vi "Facade.vi"(0 "Data In":T8={"Name"="", "Criteria"=[{"DigInput"=0, "State"=enum."Low", "Time (ms)"=0, "Name"=""}, {"DigInput"=0, "State"=enum."Low", "Time (ms)"=0, "Name"=""}], "Operators"=[], "Accumulator"={"active"=FALSE, "N"=0, "T"=0.0, "Imax"=0.0, "latency"=0.0}}, 2 "Display State In":T6, 3 "Container State":T7) -> (6 "Data Out":T8={"Name"="", "Criteria"=[{"DigInput"=0, "State"=enum."Low", "Time (ms)"=0, "Name"=""}, {"DigInput"=0, "State"=enum."Low", "Time (ms)"=0, "Name"=""}], "Operators"=[], "Accumulator"={"active"=FALSE, "N"=0, "T"=0.0, "Imax"=0.0, "latency"=0.0}}, 7 "Display State Out":T6, 8 "Action":T5)   [LabVIEW 2020, in "Input Event XCtrl.xctl"]
uses:
  Input Event XCtrl.xctl
  <vilib>/_xctls/Action.ctl
  <vilib>/_xctls/XControlSupport.lvlib
  Input Criteria Table/Input Criteria Table.xctl
  <vilib>/_xctls/Container State.ctl
  Data.vi
  State.vi
  epl-vi-lib/Utility VIs/Type Defs/Logic State.ctl
  Digital Input VIs/Tosca-Input Criterion.ctl
  Typedefs/Tosca-Accumulator.ctl
  epl-vi-lib/Utility VIs/Buttons/KCheckmarkBoolean 2.ctl
panel:
  in  "label1":string="...beginning"
  in  "label2":string="...no interval longer than"
  in  "latency":dbl caption="ms after state change..."
  in  "ms":dbl
  in  "T":dbl caption="ms..."
  in  "N":i32=2 caption="in" min=2
  in  "Accumulate":T1
  in  "Input Criteria":T4(xcontrol) caption="...is TRUE when..."
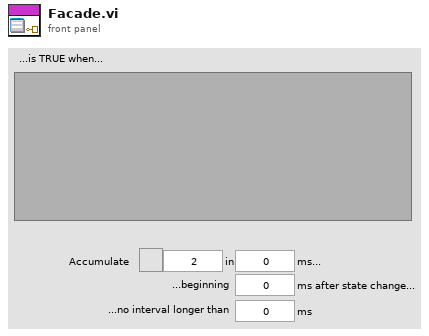
[diagram p1: front panel]
types:
  T1 = typedef "KCheckmarkBoolean 2.ctl" = bool
  T2 = typedef "Tosca-Input Criterion.ctl" = cluster{"DigInput":i32, "State":T3, "Time (ms)":i32, "Name":string}
  T3 = typedef "Logic State.ctl" = enum16{"Low", "High", "Rising", "Falling"}
  T4 = cluster{"Name":string, "Criteria":T2[], "Operators":enum16{"AND", "OR"}[]}
  T5 = typedef "XControlSupport.lvlib/Action.ctl" = cluster{"Data Changed?":bool, "State Changed?":bool, "Action Name":string}
  T6 = typedef "Input Event XCtrl.xctl/State.vi" = cluster{"Digital Inputs":string[], "Flags":string[], "action":string}
  T7 = typedef "XControlSupport.lvlib/Container State.ctl" = cluster{"Indicator?":bool, "Run Mode?":bool, " Refnum":refnum<vi>}
  T8 = typedef "Input Event XCtrl.xctl/Data.vi" = cluster{"Name":string, "Criteria":T2[], "Operators":enum16{"AND", "OR"}[], "Accumulator":T9}
  T9 = typedef "Tosca-Accumulator.ctl" = cluster{"active":bool, "N":i32, "T":dbl, "Imax":dbl, "latency":dbl}
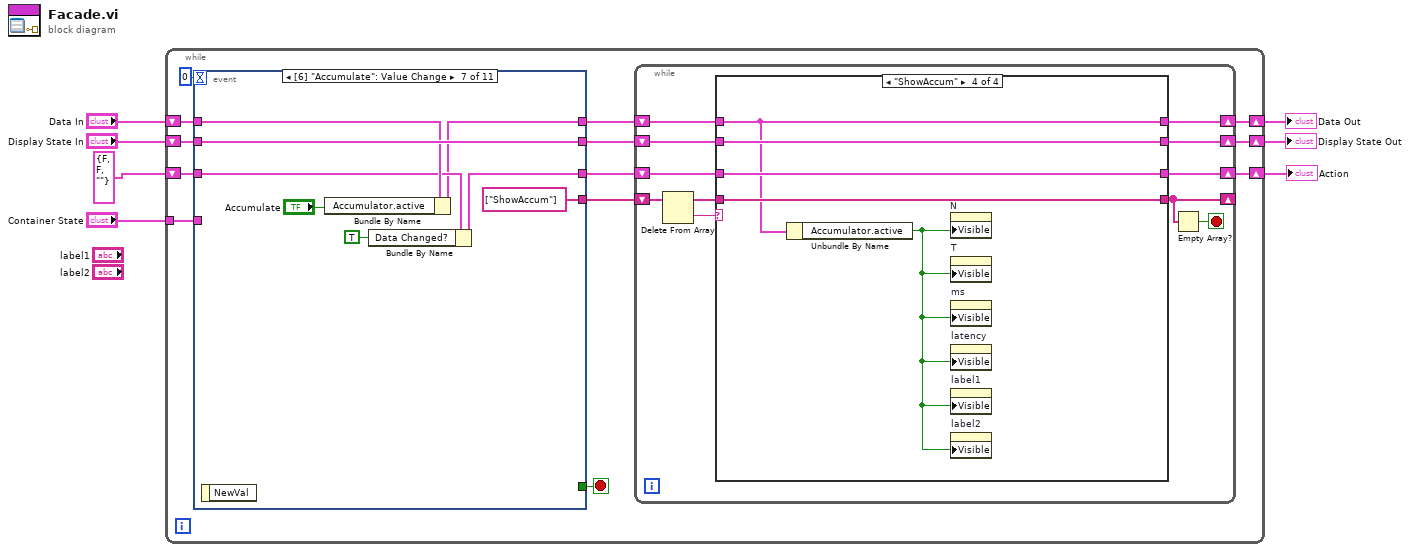
[diagram p0: block diagram]
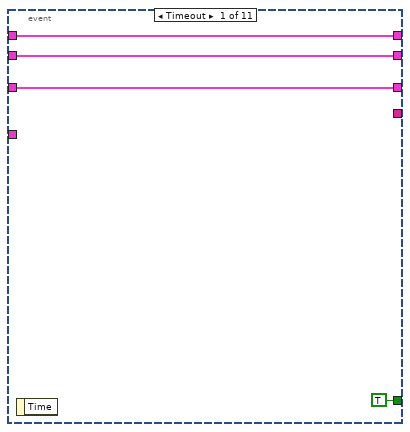
[diagram p2: hidden frame]
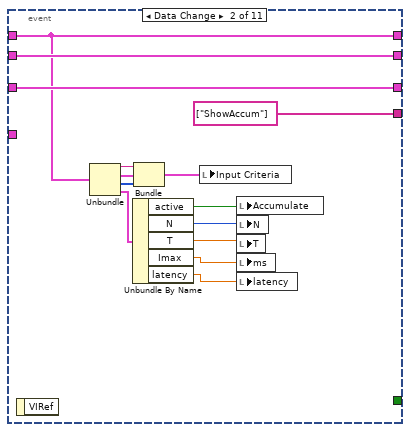
[diagram p3: hidden frame]
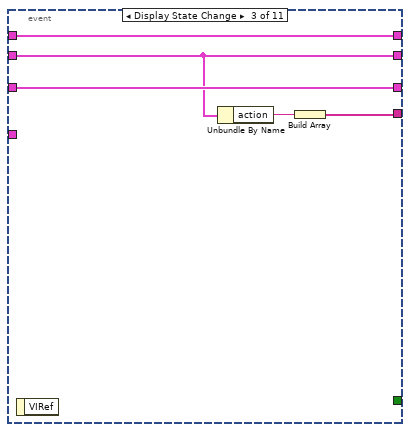
[diagram p4: hidden frame]
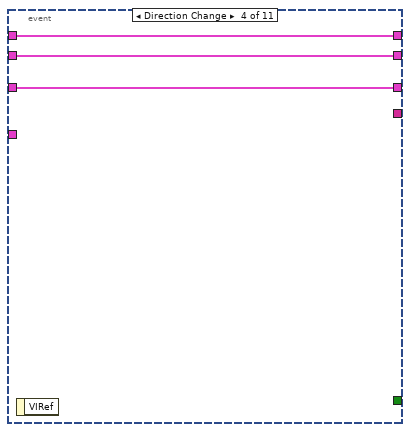
[diagram p5: hidden frame]
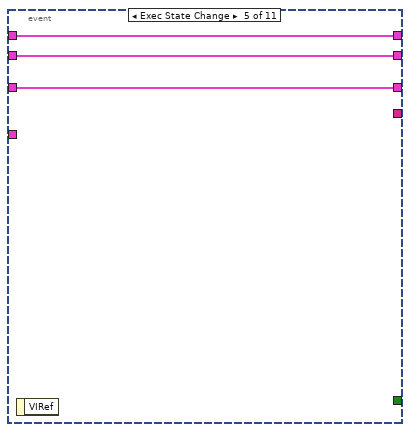
[diagram p6: hidden frame]
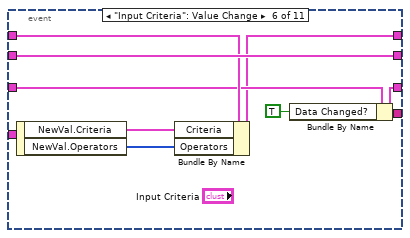
[diagram p7: hidden frame]
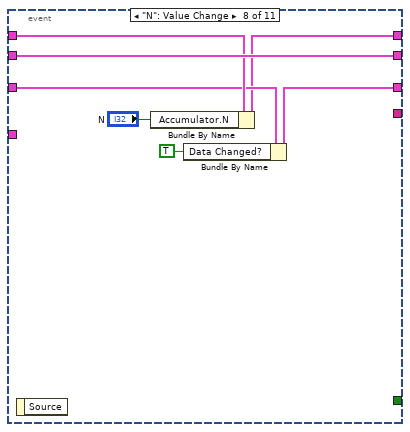
[diagram p8: hidden frame]
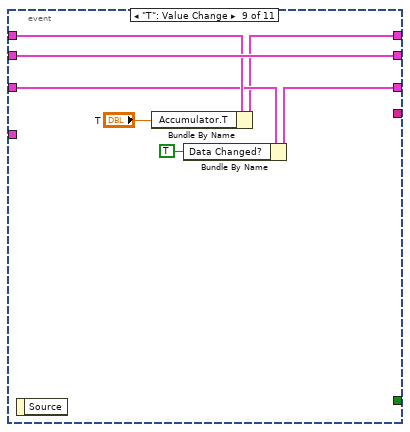
[diagram p9: hidden frame]
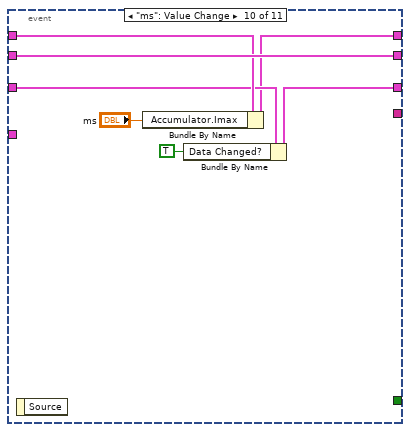
[diagram p10: hidden frame]
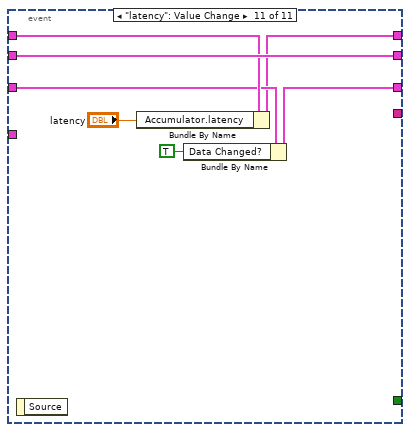
[diagram p11: hidden frame]
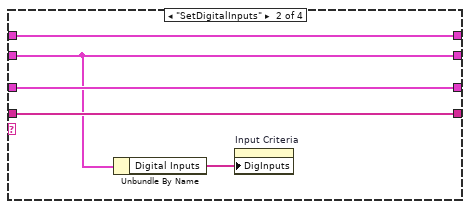
[diagram p13: hidden frame]
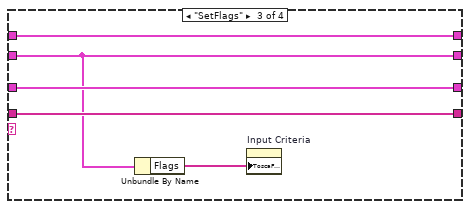
[diagram p14: hidden frame]
diagram:
  n1 = while {
    shift-right: [w8] -> w4
    shift-left: "Display State In" -> [w20]
    tunnel: "Container State" -> [w17]
    shift-right: [w10] -> w7
    shift-left: "Data In" -> [w16]
    shift-right: [w9] -> w2
    shift-left: T5 {"Data Changed?"=FALSE, "State Changed?"=FALSE, "Action Name"=""} ("Action") -> [w15]
    stop <- w19 stop-if-true
    n2 = event shown="[6] \"Accumulate\": Value Change" {
      selector: _ -> [_ _ _ _ _ _ _ _ _ _ _]
      dyn-events: _ -> [_ _ _ _ _ _ _ _ _ _ _]
      timeout: 0 -> [_ _ _ _ _ _ _ _ _ _ _]
      tunnel: w20 -> [w22 w38 w41 w46 w49 w57 w65 w72 w79 w86 w93]
      tunnel: [w22 w38 w41 w46 w49 w57 w65 w72 w79 w86 w93] -> w12
      tunnel: [TRUE _ _ _ _ _ _ _ _ _ _] -> w19
      tunnel: w17 -> [_ _ _ _ _ _ _ _ _ _ _]
      tunnel: w16 -> [w21 w31 w43 w45 w48 w56 w64 w71 w78 w85 w92]
      tunnel: [w21 w31 w43 w45 w48 w54 w61 w69 w76 w83 w90] -> w13
      tunnel: [w23 w37 w42 w44 w47 w53 w60 w68 w75 w82 w89] -> w11
      tunnel: w15 -> [w23 w37 w42 w44 w47 w55 w63 w70 w77 w84 w91]
      tunnel: [_ string[] ["ShowAccum"] w39 _ _ _ string[] ["ShowAccum"] _ _ _ _] -> w14
      event Timeout {
        n3 = event-data() -> ()  [unwired: 1 in, 1 out]
      }
      event Data Change {
        n4 = event-data() -> ()  [unwired: 1 in, 1 out]
        n5 = Unbundle(w31) -> ("Name"=w35:string, "Criteria"=w34:T2[], "Operators"=w33:enum16{"AND", "OR"}[], "Accumulator"=w32:T9)
        n6 = Unbundle By Name(w32) -> ("active"=w29:bool, "N"=w28:i32, "T"=w27:dbl, "Imax"=w26:dbl, "latency"=w25:dbl)
        n7 = Bundle("Name"=w35, "Criteria"=w34, "Operators"=w33) -> (w30:T4)  [unwired: 1 in]
        n8 = local write "Input Criteria"(w30) -> ()
        n9 = local write "Accumulate"(w29) -> ()
        n10 = local write "N"(w28) -> ()
        n11 = local write "T"(w27) -> ()
        n12 = local write "ms"(w26) -> ()
        n13 = local write "latency"(w25) -> ()
      }
      event Display State Change {
        n14 = event-data() -> ()  [unwired: 1 in, 1 out]
        n15 = Unbundle By Name(w41) -> ("action"=w40:string)
        n16 = Build Array(w40) -> (w39:string[])
      }
      event Direction Change {
        n17 = event-data() -> ()  [unwired: 1 in, 1 out]
      }
      event Exec State Change {
        n18 = event-data() -> ()  [unwired: 1 in, 1 out]
      }
      event "Input Criteria": Value Change {
        n19 = event-data() -> ("NewVal.Criteria"=w51:T2[], "NewVal.Operators"=w50:enum16{"AND", "OR"}[])  [unwired: 1 in]
        n20 = Bundle By Name(cluster=w56, "Criteria"=w51, "Operators"=w50) -> (w54:T8)
        n21 = Bundle By Name(cluster=w55, "Data Changed?"=TRUE) -> (w53:T5)
      }
      event Value Change {
        n22 = event-data() -> ()  [unwired: 1 in, 1 out]
        n23 = Bundle By Name(cluster=w64, "Accumulator.active"="Accumulate") -> (w61:T8)
        n24 = Bundle By Name(cluster=w63, "Data Changed?"=TRUE) -> (w60:T5)
      }
      event "N": Value Change {
        n25 = event-data() -> ()  [unwired: 1 in, 1 out]
        n26 = Bundle By Name(cluster=w71, "Accumulator.N"="N") -> (w69:T8)
        n27 = Bundle By Name(cluster=w70, "Data Changed?"=TRUE) -> (w68:T5)
      }
      event "T": Value Change {
        n28 = event-data() -> ()  [unwired: 1 in, 1 out]
        n29 = Bundle By Name(cluster=w78, "Accumulator.T"="T") -> (w76:T8)
        n30 = Bundle By Name(cluster=w77, "Data Changed?"=TRUE) -> (w75:T5)
      }
      event "ms": Value Change {
        n31 = event-data() -> ()  [unwired: 1 in, 1 out]
        n32 = Bundle By Name(cluster=w85, "Accumulator.Imax"="ms") -> (w83:T8)
        n33 = Bundle By Name(cluster=w84, "Data Changed?"=TRUE) -> (w82:T5)
      }
      event "latency": Value Change {
        n34 = event-data() -> ()  [unwired: 1 in, 1 out]
        n35 = Bundle By Name(cluster=w92, "Accumulator.latency"="latency") -> (w90:T8)
        n36 = Bundle By Name(cluster=w91, "Data Changed?"=TRUE) -> (w89:T5)
      }
    }
    n37 = while {
      shift-right: [w101] -> _
      shift-left: w14 -> [w104]
      shift-right: [w98] -> w10
      shift-left: w13 -> [w99]
      shift-right: [w97] -> w8
      shift-left: w12 -> [w96]
      shift-right: [w95] -> w9
      shift-left: w11 -> [w94]
      stop <- w100 stop-if-true
      n38 = Delete From Array(array=w104) -> (deleted portion=w102:string, array with subset deleted=w103:string[])  [unwired: 2 in]
      n39 = case shown="\"ShowAccum\"" w102 {
        tunnel: w103 -> [w108 w113 w118 w123]
        tunnel: [w108 w113 w118 w123] -> w101
        tunnel: w99 -> [w107 w112 w117 w120]
        tunnel: [w107 w112 w117 w120] -> w98
        tunnel: [w106 w110 w115 w122] -> w97
        tunnel: w96 -> [w106 w110 w115 w122]
        tunnel: [w105 w111 w116 w121] -> w95
        tunnel: w94 -> [w105 w111 w116 w121]
        frame "", Default {
        }
        frame "SetDigitalInputs" {
          n40 = Unbundle By Name(w110) -> ("Digital Inputs"=w109:string[])
          n41 = property on="Input Criteria" class="Input Criteria Table (strict)"("DigInputs"=w109) -> ()  [unwired: 2 in, 2 out]
        }
        frame "SetFlags" {
          n42 = Unbundle By Name(w115) -> ("Flags"=w114:string[])
          n43 = property on="Input Criteria" class="Input Criteria Table (strict)"("ToscaFlags"=w114) -> ()  [unwired: 2 in, 2 out]
        }
        frame "ShowAccum" {
          n44 = Unbundle By Name(w120) -> ("Accumulator.active"=w119:bool)
          n45 = property on="N" class="DigNum (strict)"("Visible"=w119) -> ()  [unwired: 2 in, 2 out]
          n46 = property on="T" class="DigNum (strict)"("Visible"=w119) -> ()  [unwired: 2 in, 2 out]
          n47 = property on="ms" class="DigNum (strict)"("Visible"=w119) -> ()  [unwired: 2 in, 2 out]
          n48 = property on="latency" class="DigNum (strict)"("Visible"=w119) -> ()  [unwired: 2 in, 2 out]
          n49 = property on="label1" class="Str"("Visible"=w119) -> ()  [unwired: 2 in, 2 out]
          n50 = property on="label2" class="Str"("Visible"=w119) -> ()  [unwired: 2 in, 2 out]
        }
      }
      n51 = Empty Array?(array=w101) -> (empty?=w100:bool)
    }
  }
  "Display State Out" <- w4
  "Data Out" <- w7
  "Action" <- w2
